vi "main.vi"() -> ()   [LabVIEW 2024]
uses:
  Downloads/globalVar.vi
panel:
  in  "Array 2":bool[][](array[boolean])
  in  "stop":bool
  in  "OK Button 2":bool
  in  "OK Button":bool
  in  "stop 2":bool
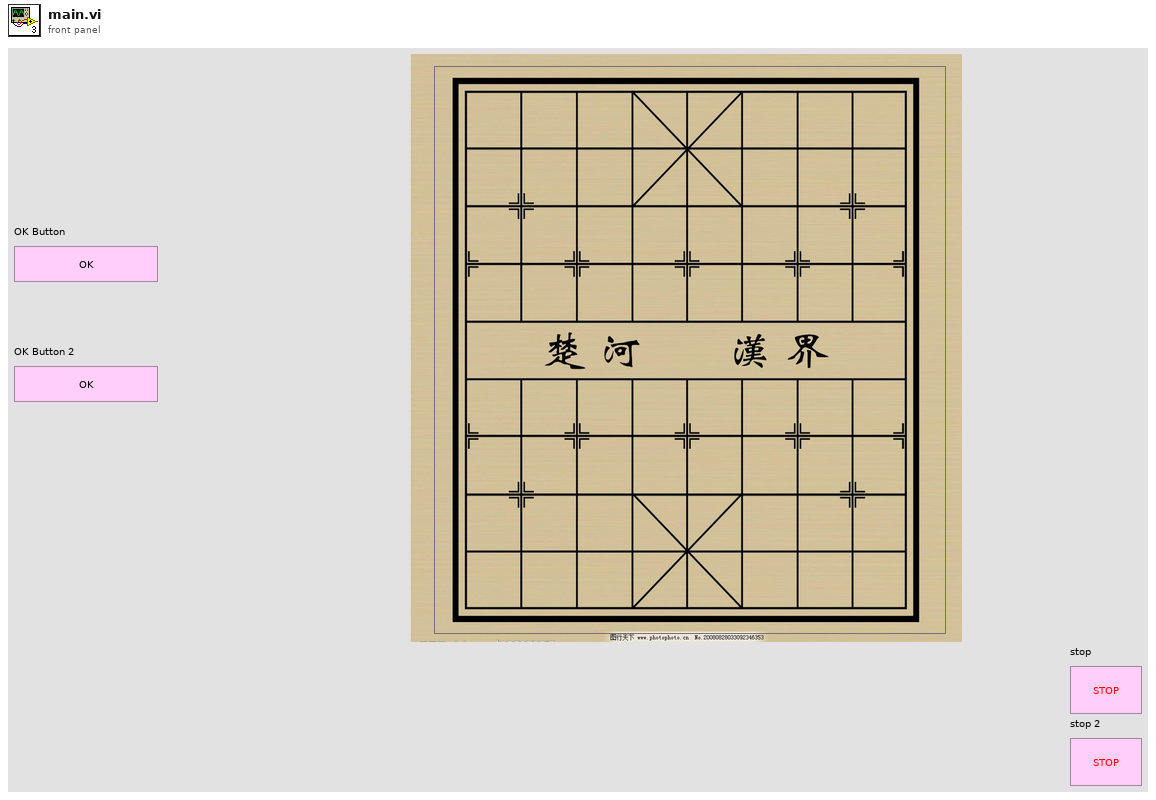
[diagram p1: front panel]
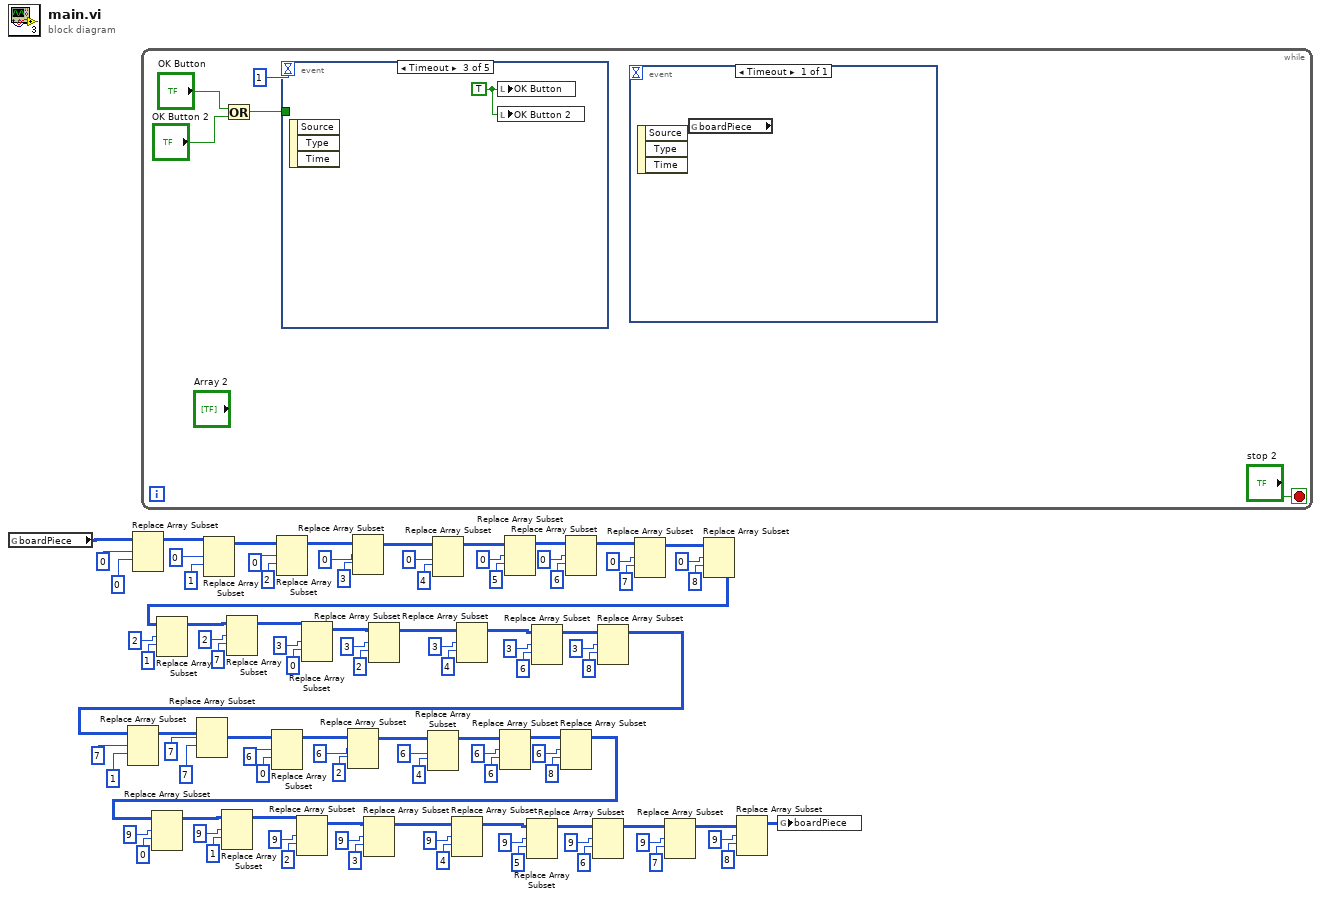
[diagram p0: block diagram]
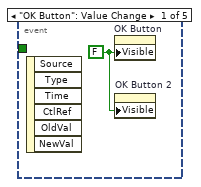
[diagram p2: hidden frame]
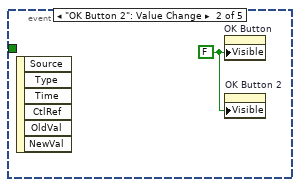
[diagram p3: hidden frame]
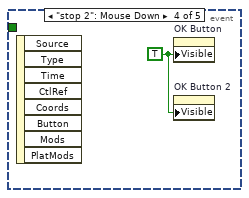
[diagram p4: hidden frame]
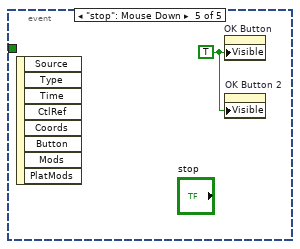
[diagram p5: hidden frame]
diagram:
  n1 = global read "globalVar.vi" "boardPiece"() -> (w72:i32[][])
  n2 = Replace Array Subset(array=w72, index (row)=0, index (col)=0) -> (w71:i32[][])  [unwired: 1 in]
  n3 = while {
    stop <- "stop 2" stop-if-true
    n4 = Or(x="OK Button", y="OK Button 2") -> (x .or. y?=w102:bool)
    n5 = event shown="[2] Timeout" {
      selector: _ -> [_ _ _ _ _]
      dyn-events: _ -> [_ _ _ _ _]
      timeout: 1 -> [_ _ _ _ _]
      tunnel: w102 -> [_ _ _ _ _]
      event "OK Button": Value Change {
        w103 = FALSE ("Visible")
        n6 = event-data() -> ()  [unwired: 1 in, 6 out]
        n7 = property on="OK Button" class="Bool (strict)"("Visible"=w103) -> ()  [unwired: 2 in, 2 out]
        n8 = property on="OK Button 2" class="Bool (strict)"("Visible"=w103) -> ()  [unwired: 2 in, 2 out]
      }
      event "OK Button 2": Value Change {
        w104 = FALSE ("Visible")
        n9 = event-data() -> ()  [unwired: 1 in, 6 out]
        n10 = property on="OK Button" class="Bool (strict)"("Visible"=w104) -> ()  [unwired: 2 in, 2 out]
        n11 = property on="OK Button 2" class="Bool (strict)"("Visible"=w104) -> ()  [unwired: 2 in, 2 out]
      }
      event Timeout {
        w105 = TRUE ("Visible")
        n12 = event-data() -> ()  [unwired: 1 in, 3 out]
        n13 = local write "OK Button"(w105) -> ()
        n14 = local write "OK Button 2"(w105) -> ()
      }
      event "stop 2": Mouse Down {
        w106 = TRUE ("Visible")
        n15 = event-data() -> ()  [unwired: 1 in, 8 out]
        n16 = property on="OK Button" class="Bool (strict)"("Visible"=w106) -> ()  [unwired: 2 in, 2 out]
        n17 = property on="OK Button 2" class="Bool (strict)"("Visible"=w106) -> ()  [unwired: 2 in, 2 out]
      }
      event "stop": Mouse Down {
        w107 = TRUE ("Visible")
        n18 = event-data() -> ()  [unwired: 1 in, 8 out]
        n19 = property on="OK Button" class="Bool (strict)"("Visible"=w107) -> ()  [unwired: 2 in, 2 out]
        n20 = property on="OK Button 2" class="Bool (strict)"("Visible"=w107) -> ()  [unwired: 2 in, 2 out]
      }
    }
    n21 = event shown="[0] Timeout" {
      selector: _ -> [_]
      dyn-events: _ -> [_]
      timeout: _ -> [_]
      event Timeout {
        n22 = event-data() -> ()  [unwired: 1 in, 3 out]
        n23 = global read "globalVar.vi" "boardPiece"() -> ()  [unwired: 1 out]
      }
    }
  }
  n24 = Replace Array Subset(array=w71, index (row)=0, index (col)=1) -> (w93:i32[][])  [unwired: 1 in]
  n25 = Replace Array Subset(array=w93, index (row)=0, index (col)=2) -> (w91:i32[][])  [unwired: 1 in]
  n26 = Replace Array Subset(array=w91, index (row)=0, index (col)=3) -> (w89:i32[][])  [unwired: 1 in]
  n27 = Replace Array Subset(array=w89, index (row)=0, index (col)=4) -> (w85:i32[][])  [unwired: 1 in]
  n28 = Replace Array Subset(array=w85, index (row)=0, index (col)=5) -> (w81:i32[][])  [unwired: 1 in]
  n29 = Replace Array Subset(array=w81, index (row)=0, index (col)=6) -> (w76:i32[][])  [unwired: 1 in]
  n30 = Replace Array Subset(array=w76, index (row)=0, index (col)=7) -> (w75:i32[][])  [unwired: 1 in]
  n31 = Replace Array Subset(array=w75, index (row)=0, index (col)=8) -> (w66:i32[][])  [unwired: 1 in]
  n32 = Replace Array Subset(array=w66, index (row)=2, index (col)=1) -> (w65:i32[][])  [unwired: 1 in]
  n33 = Replace Array Subset(array=w65, index (row)=2, index (col)=7) -> (w54:i32[][])  [unwired: 1 in]
  n34 = Replace Array Subset(array=w54, index (row)=3, index (col)=0) -> (w53:i32[][])  [unwired: 1 in]
  n35 = Replace Array Subset(array=w53, index (row)=3, index (col)=2) -> (w52:i32[][])  [unwired: 1 in]
  n36 = Replace Array Subset(array=w52, index (row)=3, index (col)=4) -> (w51:i32[][])  [unwired: 1 in]
  n37 = Replace Array Subset(array=w51, index (row)=3, index (col)=6) -> (w50:i32[][])  [unwired: 1 in]
  n38 = Replace Array Subset(array=w50, index (row)=3, index (col)=8) -> (w10:i32[][])  [unwired: 1 in]
  n39 = Replace Array Subset(array=w10, index (row)=7, index (col)=1) -> (w29:i32[][])  [unwired: 1 in]
  n40 = Replace Array Subset(array=w29, index (row)=7, index (col)=7) -> (w15:i32[][])  [unwired: 1 in]
  n41 = Replace Array Subset(array=w15, index (row)=6, index (col)=0) -> (w17:i32[][])  [unwired: 1 in]
  n42 = Replace Array Subset(array=w17, index (row)=6, index (col)=2) -> (w19:i32[][])  [unwired: 1 in]
  n43 = Replace Array Subset(array=w19, index (row)=6, index (col)=4) -> (w23:i32[][])  [unwired: 1 in]
  n44 = Replace Array Subset(array=w23, index (row)=6, index (col)=6) -> (w27:i32[][])  [unwired: 1 in]
  n45 = Replace Array Subset(array=w27, index (row)=6, index (col)=8) -> (w8:i32[][])  [unwired: 1 in]
  n46 = Replace Array Subset(array=w8, index (row)=9, index (col)=0) -> (w34:i32[][])  [unwired: 1 in]
  n47 = Replace Array Subset(array=w34, index (row)=9, index (col)=1) -> (w45:i32[][])  [unwired: 1 in]
  n48 = Replace Array Subset(array=w45, index (row)=9, index (col)=2) -> (w46:i32[][])  [unwired: 1 in]
  n49 = Replace Array Subset(array=w46, index (row)=9, index (col)=3) -> (w47:i32[][])  [unwired: 1 in]
  n50 = Replace Array Subset(array=w47, index (row)=9, index (col)=4) -> (w48:i32[][])  [unwired: 1 in]
  n51 = Replace Array Subset(array=w48, index (row)=9, index (col)=5) -> (w49:i32[][])  [unwired: 1 in]
  n52 = Replace Array Subset(array=w49, index (row)=9, index (col)=6) -> (w3:i32[][])  [unwired: 1 in]
  n53 = Replace Array Subset(array=w3, index (row)=9, index (col)=7) -> (w2:i32[][])  [unwired: 1 in]
  n54 = Replace Array Subset(array=w2, index (row)=9, index (col)=8) -> (w1:i32[][])  [unwired: 1 in]
  n55 = global write "globalVar.vi" "boardPiece"(w1) -> ()
